vi "S2DS_ExitCondition.vi"(7 "Scan parameters in":T1 {"Y data taking" items=["in both direction", "in up direction only", "in down direction only"]; "X data taking" items=["in both direction", "in up direction only", "in down direction only"]}, 9 "Buffer length":i32) -> (3 "Yes, exit.":bool)   [LabVIEW 2025]
uses:
  TYPE DEFS/S2DS_Sweep Info.ctl
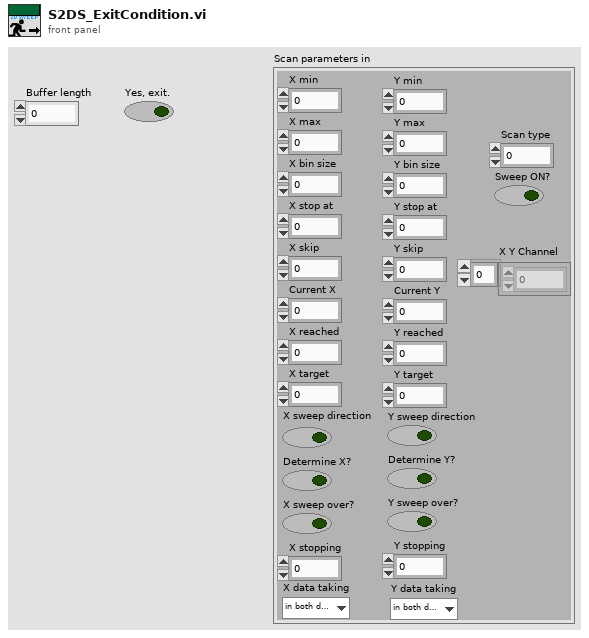
[diagram p1: front panel]
types:
  T1 = typedef "S2DS_Sweep Info.ctl" = cluster{"X min":ext, "X max":dbl, "Y min":dbl, "Y max":dbl, "X bin size":dbl, "Y bin size":dbl, "X stop at":dbl, "Y stop at":dbl, "X skip":u64, "Y skip":u64, "Current X":dbl, "Current Y":dbl, "X reached":i32, "Y reached":i32, "X target":dbl, "Y target":dbl, "Sweep ON?":bool, "X sweep direction":bool, "Y sweep direction":bool, "Determine X?":bool, "Determine Y?":bool, "X sweep over?":bool, "Y sweep over?":bool, "Scan type":i32, "X stopping":i32, "Y stopping":i32, "X Y Channel":u16[], "X data taking":u16, "Y data taking":u16}
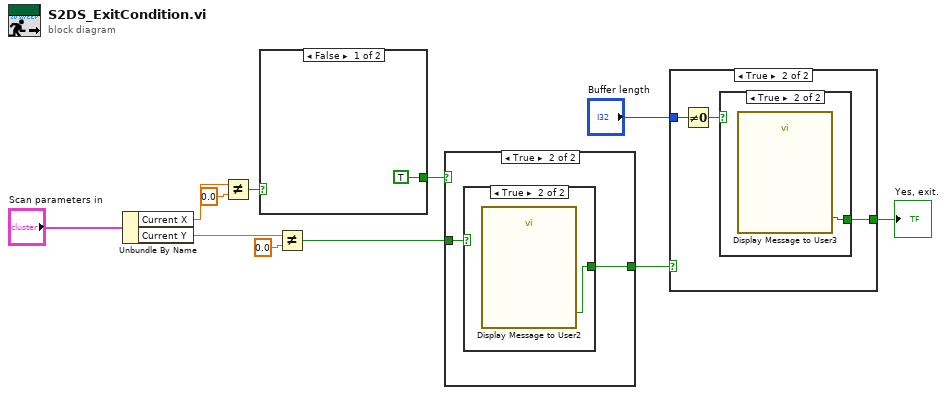
[diagram p0: block diagram]
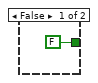
[diagram p2: hidden frame]
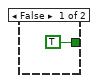
[diagram p3: hidden frame]
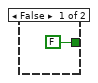
[diagram p4: hidden frame]
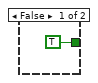
[diagram p5: hidden frame]
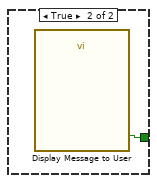
[diagram p6: hidden frame]
diagram:
  n1 = Unbundle By Name("Scan parameters in") -> ("Current X"=w8:dbl, "Current Y"=w7:dbl)
  n2 = Not Equal?(x=w8, y=0.0) -> (x != y?=w6:bool)
  n3 = case shown="False" w6 {
    tunnel: [TRUE w13] -> w3
    frame False {
    }
    frame True {
      n4 = call "Display Message to User"() -> ("Yes, exit."=w13:bool)  [unwired: 10 in, 1 out]
    }
  }
  n5 = Not Equal?(x=w7, y=0.0) -> (x != y?=w2:bool)
  n6 = case shown="True" w3 {
    tunnel: [FALSE w16] -> w1
    tunnel: w2 -> [_ w15]
    frame False {
    }
    frame True {
      n7 = case shown="True" w15 {
        tunnel: [TRUE w18] -> w16
        frame False {
        }
        frame True {
          n8 = call "Display Message to User2"() -> ("Yes, exit."=w18:bool)  [unwired: 10 in, 1 out]
        }
      }
    }
  }
  n9 = case shown="True" w1 {
    tunnel: [FALSE w21] -> w10
    tunnel: "Buffer length" -> [_ w20]
    frame False {
    }
    frame True {
      n10 = Not Equal To 0?(x=w20) -> (x != 0?=w22:bool)
      n11 = case shown="True" w22 {
        tunnel: [TRUE w24] -> w21
        frame False {
        }
        frame True {
          n12 = call "Display Message to User3"() -> ("Yes, exit."=w24:bool)  [unwired: 10 in, 1 out]
        }
      }
    }
  }
  "Yes, exit." <- w10
